vi "Size of Variant Array.vi"(8 "error in (no error)":errorcluster, 11 "LabVIEW Array In":variant) -> (0 "error out":errorcluster, 2 "Size of Array":u32)   [LabVIEW 2014, in "i3-json.lvlib"]
doc: "Returns the size of a Variant array"
uses:
  i3-json.lvlib
  <vilib>/Utility/VariantDataType/VariantType.lvlib
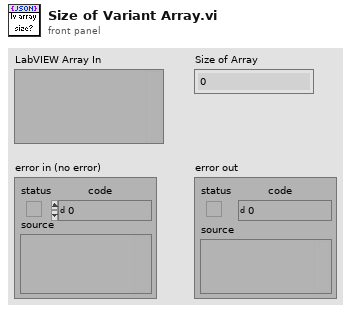
[diagram p1: front panel]
types:
  T1 = typedef "VariantType.lvlib/MemoryInfo.ctl" = cluster{"Type":T2, "Size":u32}
  T2 = typedef "VariantType.lvlib/MemoryType.ctl" = enum16{"Variable", "Fixed", "Bounded"}
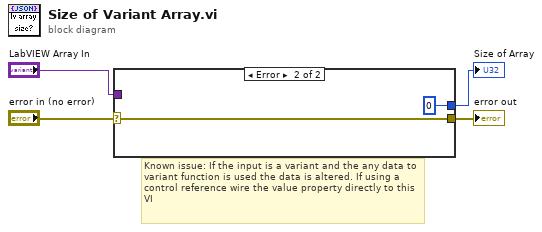
[diagram p0: block diagram]
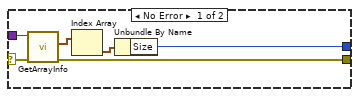
[diagram p2: hidden frame]
diagram:
  # "Known issue: If the input is a variant and the any data to variant function is used the data is altered. If using a control reference wire the value property directly to this VI"
  n1 = case shown="Error" "error in (no error)" {
    selector: "error in (no error)" -> [w5 w12]
    tunnel: "LabVIEW Array In" -> [w8 _]
    tunnel: [w6 w12] -> w2
    tunnel: [w9 u32 0 ("number")] -> w1
    frame No Error {
      n2 = call <vilib>:"GetArrayInfo.vi"("error in (no error)"=w5, "Variant"=w8) -> ("error out"=w6:errorcluster, "Array Lengths"=w7:T1[])  [unwired: 6 in, 2 out]
      n3 = Index Array(array=w7) -> (element=w10:T1)  [unwired: 1 in]
      n4 = Unbundle By Name(w10) -> ("Size"=w9:u32)
    }
    frame Error {
    }
  }
  "error out" <- w2
  "Size of Array" <- w1
